vi "Get Mean Oblique Ecliptic.vi"(11 "Julian Century":dbl) -> (3 "Mean Obique Ecliptic Longitude":dbl)   [LabVIEW 2014, in "Solar Calculations.lvlib"]
uses:
  Solar Calculations.lvlib
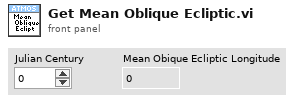
[diagram p1: front panel]
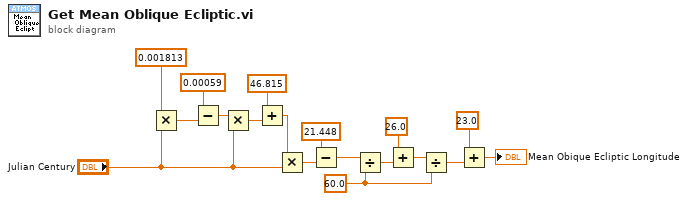
[diagram p0: block diagram]
diagram:
  w14 = 60.0 ("y")
  n1 = Multiply(x=0.001813, y="Julian Century") -> (x*y=w3:dbl)
  n2 = Subtract(x=0.00059, y=w3) -> (x-y=w4:dbl)
  n3 = Multiply(x=w4, y="Julian Century") -> (x*y=w5:dbl)
  n4 = Add(x=46.815, y=w5) -> (x+y=w7:dbl)
  n5 = Multiply(x=w7, y="Julian Century") -> (x*y=w8:dbl)
  n6 = Subtract(x=21.448, y=w8) -> (x-y=w10:dbl)
  n7 = Divide(x=w10, y=w14) -> (x/y=w11:dbl)
  n8 = Add(x=26.0, y=w11) -> (x+y=w13:dbl)
  n9 = Divide(x=w13, y=w14) -> (x/y=w15:dbl)
  n10 = Add(x=23.0, y=w15) -> (x+y=→"Mean Obique Ecliptic Longitude":dbl)
